vi "Read relay name.vi"(8 "error in (no error)":errorcluster, 11 "Relay in":refnum<class "Relay.lvclass">) -> (0 "error out":errorcluster, 2 "name":string, 3 "Relay out":refnum<class "Relay.lvclass">)   [LabVIEW 2016, in "SLSC Switch.lvlib" / "Relay.lvclass"]
uses:
  Relay.lvclass
  Relay.lvclass/Relay.ctl
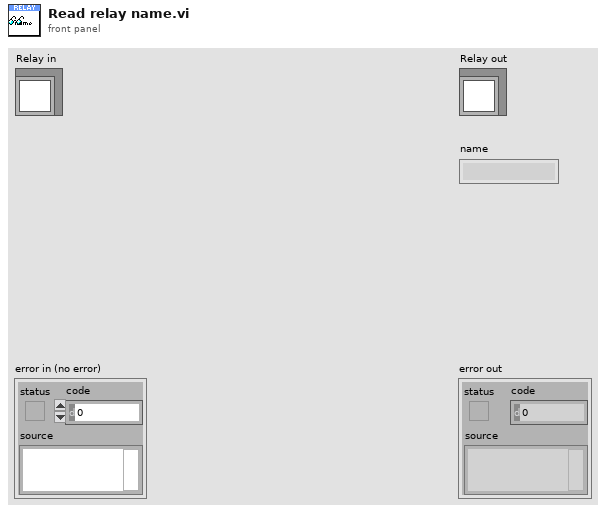
[diagram p1: front panel]
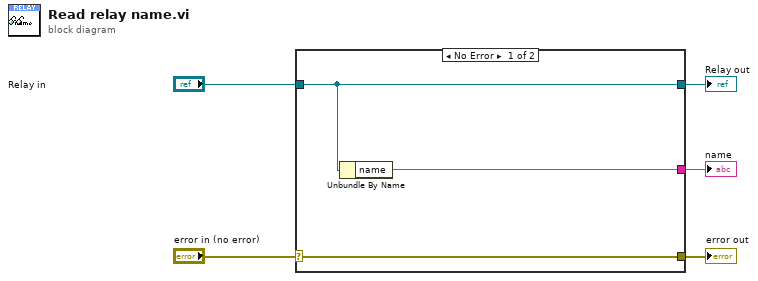
[diagram p0: block diagram]
diagram:
  n1 = case shown="No Error" "error in (no error)" {
    selector: "error in (no error)" -> [w8 w9]
    tunnel: [w8 w9] -> w4
    tunnel: [w7 w10] -> w2
    tunnel: "Relay in" -> [w7 w10]
    tunnel: [w6 _] -> w1
    frame No Error {
      n2 = Unbundle By Name(w7) -> ("name"=w6:string)
    }
    frame Error {
    }
  }
  "error out" <- w4
  "Relay out" <- w2
  "name" <- w1
